vi "ErrorHandler.GetBroadcasts.vi"(11 "NewTemplate in":refnum<class "ErrorHandler.lvclass">) -> (2 "TemplateModule":cluster{"Broadcasts":T1, "Broadcasts":T2}, 3 "NewTemplate out":refnum<class "ErrorHandler.lvclass">)   [LabVIEW 2024, in "ErrorHandler.lvclass"]
uses:
  ErrorHandler.lvclass/ErrorHandler.ctl
  ErrorHandler.lvclass
  JQMHCore/Module/RQMHModule.lvclass
  JQMHCore/Shared/Died.ctl
  JQMHCore/Shared/RQMHShared.lvlib
  JQMHCore/Module/StandardBroadcasts.ctl
  Stopped.ctl
  Broadcast Events--cluster.ctl
  JQMHCore/Module/Started.ctl
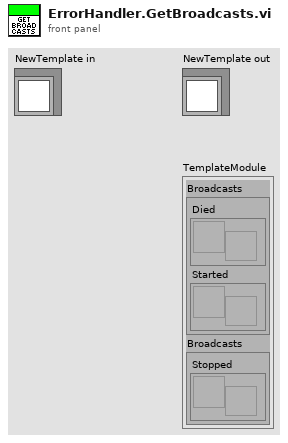
[diagram p1: front panel]
types:
  T1 = typedef "RQMHModule.lvclass/StandardBroadcasts.ctl" = cluster{"Died":refnum<user-event>, "Started":refnum<user-event>}
  T2 = typedef "ErrorHandler.lvclass/Broadcast Events--cluster.ctl" = cluster{"Stopped":refnum<user-event>}
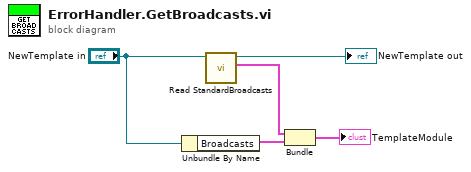
[diagram p0: block diagram]
diagram:
  n1 = Unbundle By Name("NewTemplate in") -> ("Broadcasts"=w5:T2)
  n2 = call "Read StandardBroadcasts.vi"("JQMHCore in"="NewTemplate in") -> ("Broadcasts"=w4:T1, "JQMHCore out"=→"NewTemplate out":refnum<class "ErrorHandler.lvclass">)  [unwired: 8 in, 1 out]
  n3 = Bundle("Broadcasts"=w4, "Broadcasts"=w5) -> (→"TemplateModule":cluster{"Broadcasts":T1, "Broadcasts":T2})  [unwired: 1 in]
